vi "WSVCAP SHL Host LL Interface Core.vi"(0 "Message In":string, 11 "error in":errorcluster, 12 "Log (T)":bool=TRUE, 13 "Function":T5, 14 "FPGA":T1) -> (3 "System":T2={"Settings"={"I2C Slave Address"=144, "I2C Clock Rate (Hz)"=20.0, "SPI Clock Rate (Hz)"=50000.0, "RFFE Slave Address"=255, "RFFE Clock Rate (Hz)"=20.0, "Simulate FPGA"=TRUE, "C1 Cap DAC Default"=165, "C2 Cap DAC Default"=165, "C3 Cap DAC Default"=134}, "FPGA Resource"="", "Online"=FALSE, "I2C Wait Ticks"=0, "SPI Wait Ticks"=0, "RFFE Wait Ticks"=0, "FPGA VI Reference (FPGA Mode)"=refnum, "FPGA VI Reference (Sim Mode)"=refnum} {"Settings"."C3 Cap DAC Default" format="0x%02x"; "Settings"."C2 Cap DAC Default" format="0x%02x"; "Settings"."C1 Cap DAC Default" format="0x%02x"; "Settings"."RFFE Clock Rate (Hz)" format="%.0f Hz"; "Settings"."RFFE Slave Address" format="0x%02x"; "Settings"."I2C Clock Rate (Hz)" format="%.0f Hz"; "Settings"."SPI Clock Rate (Hz)" format="%.0f Hz"; "Settings"."I2C Slave Address" format="0x%02x"}, 4 "Message Out":string, 15 "error out":errorcluster)   [LabVIEW 2012]
uses:
  Type Defs/WSVCAP SHL Function Enum.ctl
  Type Defs/WSVCAP SHL Core System Cluster.ctl
  Type Defs/WSVCAP SHL I2C Settings Cluster.ctl
  Type Defs/WSVCAP SHL FPGA VI Reference.ctl
  Type Defs/WSVCAP SHL I2C FPGA Enum.ctl
  user.lib/Configuration Files/Type Defs/CFG File Operation Enum.ctl
  Type Defs/WSVCAP SHL Top Level Control Operation Enum.ctl
  Type Defs/WSVCAP SHL Top Level Control Enum.ctl
  <vilib>/FPGAPlugInAG/PXI-7813R/niLvFpga_Open_PXI-7813R.vi
  <vilib>/FPGAPlugInAG/PXI-7813R/niLvFpga_Reset_PXI-7813R.vi
  <vilib>/FPGAPlugInAG/PXI-7813R/niLvFpga_Run_PXI-7813R.vi
  <vilib>/FPGAPlugInAG/PXI-7813R/niLvFpga_Abort_PXI-7813R.vi
  <vilib>/FPGAPlugInAG/PXI-7813R/niLvFpga_Close_PXI-7813R.vi
  <vilib>/rvi/interface/nirviOpenFPGA/nirviOpenFPGA.xnode
  FPGA Bitfiles/WSVCAPShell_WiSpryFPGA1_WSVCAPSHLFPGATLT_acCLp6kl0Ls.lvbitx
  <vilib>/rvi/interface/nirviMethod/nirviMethod.xnode
  <vilib>/rvi/interface/nirviCloseFPGA/nirviCloseFPGA.xnode
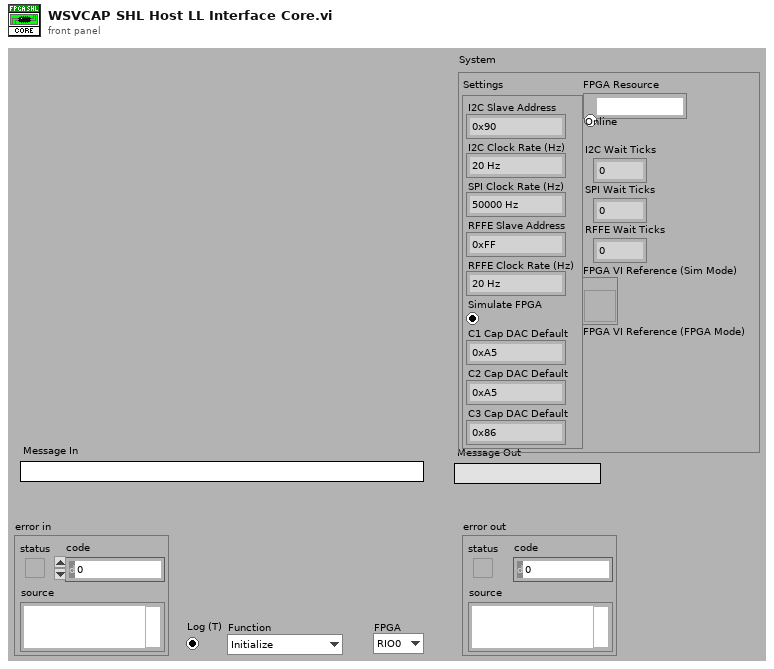
[diagram p1: front panel]
types:
  T1 = typedef "WSVCAP SHL I2C FPGA Enum.ctl" = enum16{"RIO0", "RIO1"}
  T2 = typedef "WSVCAP SHL Core System Cluster.ctl" = cluster{"Settings":T3, "FPGA Resource":tag, "Online":bool, "I2C Wait Ticks":u32, "SPI Wait Ticks":u32, "RFFE Wait Ticks":u32, "FPGA VI Reference (FPGA Mode)":T4, "FPGA VI Reference (Sim Mode)":refnum<vi>}
  T3 = typedef "WSVCAP SHL I2C Settings Cluster.ctl" = cluster{"I2C Slave Address":u8, "I2C Clock Rate (Hz)":dbl, "SPI Clock Rate (Hz)":dbl, "RFFE Slave Address":u8, "RFFE Clock Rate (Hz)":dbl, "Simulate FPGA":bool, "C1 Cap DAC Default":u8, "C2 Cap DAC Default":u8, "C3 Cap DAC Default":u8}
  T4 = typedef "WSVCAP SHL FPGA VI Reference.ctl" = refnum<k20>
  T5 = typedef "WSVCAP SHL Function Enum.ctl" = enum16{"Initialize", "Configure I2C", "Configure RFFE", "Write I2C", "Read I2C", "Write RFFE", "Read RFFE", "Start RFFE Cycle", "Stop RFFE Cycle", "Get Status", "Close"}
  T6 = typedef "WSVCAP SHL Top Level Control Operation Enum.ctl" = enum16{"Initialize", "Set Control", "Read Control", "Close"}
  T7 = typedef "CFG File Operation Enum.ctl" = enum16{"Read", "Write", "Copy", "Edit"}
  T8 = enum32{"Invalid", "Standard", "Closed", "Hidden", "Minimized", "Maximized"}
  T9 = typedef "WSVCAP SHL Top Level Control Enum.ctl" = enum16{"Start", "Cmd", "Transaction", "Wait Ticks", "Socket Mask", "UUT Set", "Slave Address", "Sub Address", "Bytes to Write", "Bytes to Read", "Write Data", "Write Flag", "Read Data", "Read Flag", "Ack Read", "Read Status Flag", "Ack Read Status", "Status", "Cycle Count", "Stop Cycle", "Exit"}
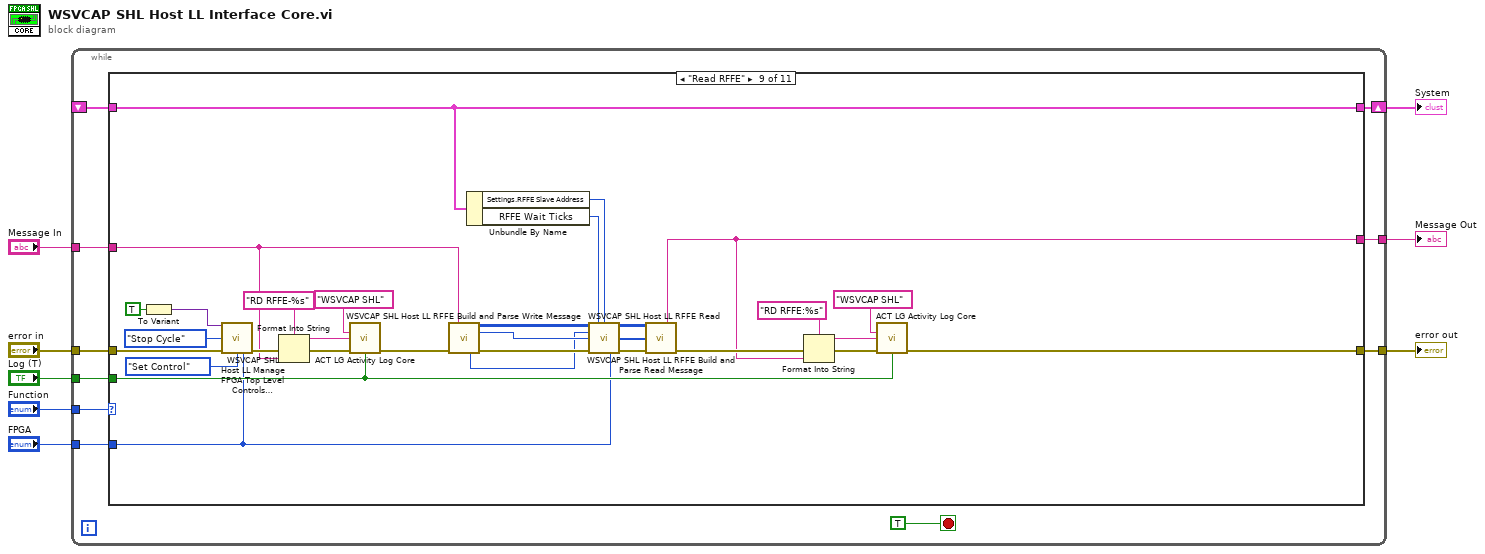
[diagram p0: block diagram]
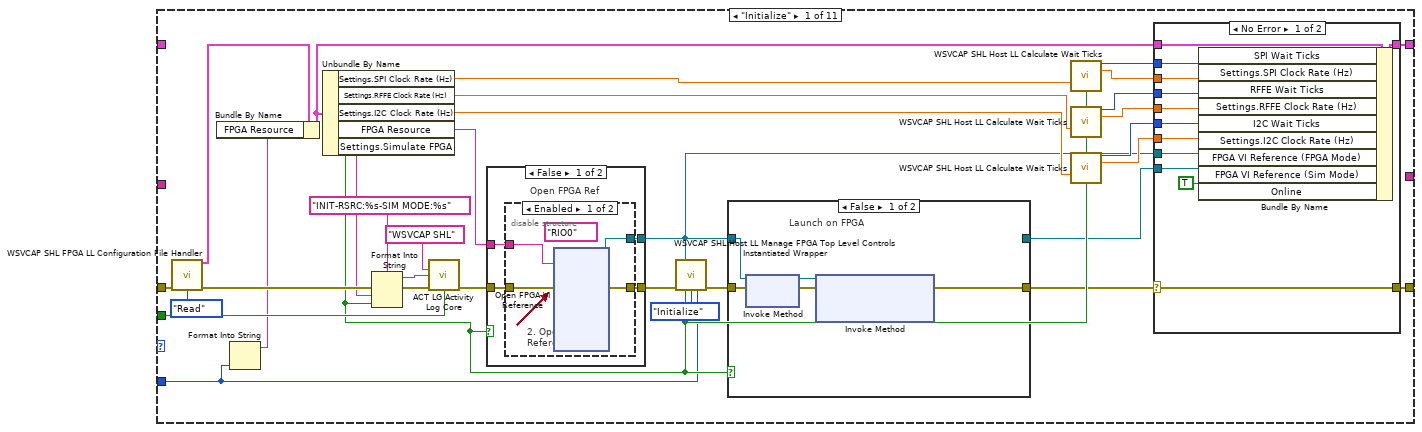
[diagram p2: hidden frame]
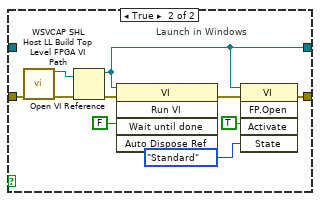
[diagram p5: hidden frame]
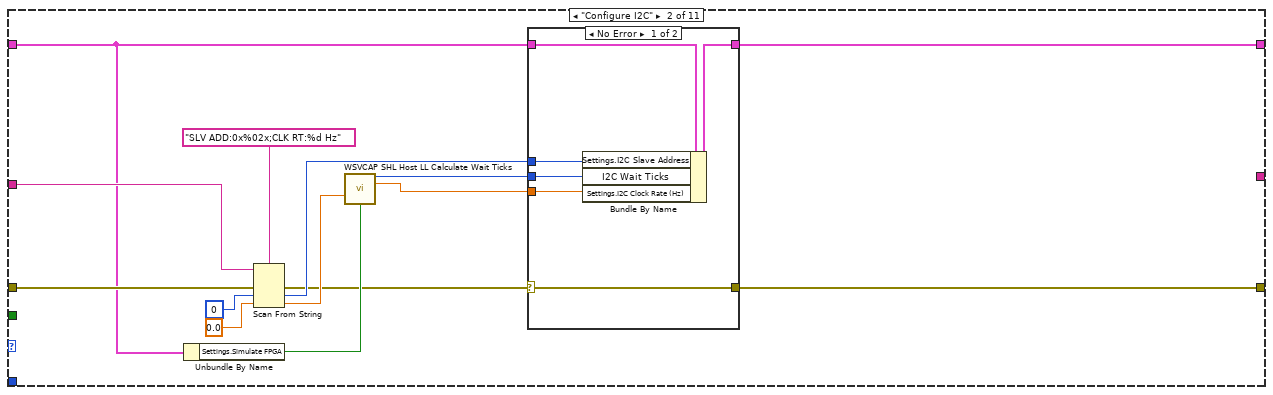
[diagram p7: hidden frame]
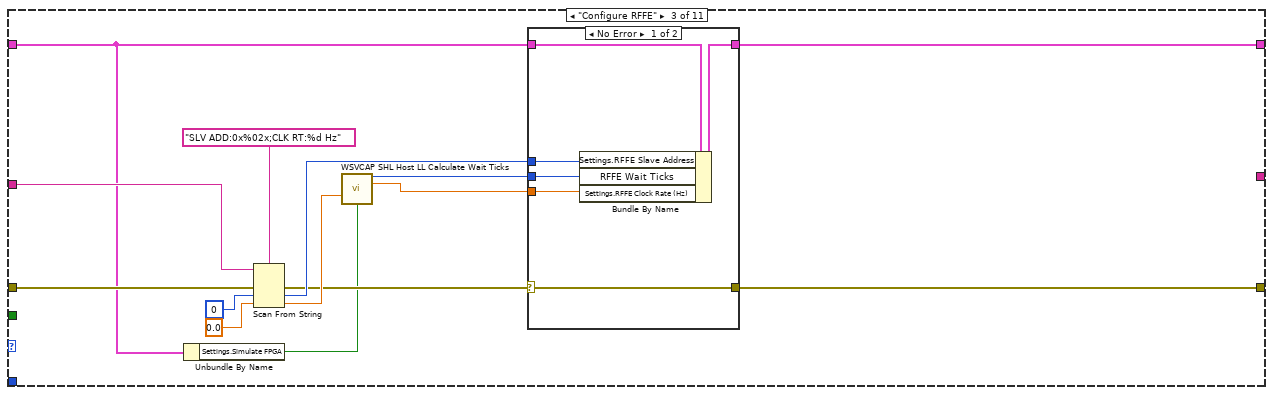
[diagram p9: hidden frame]
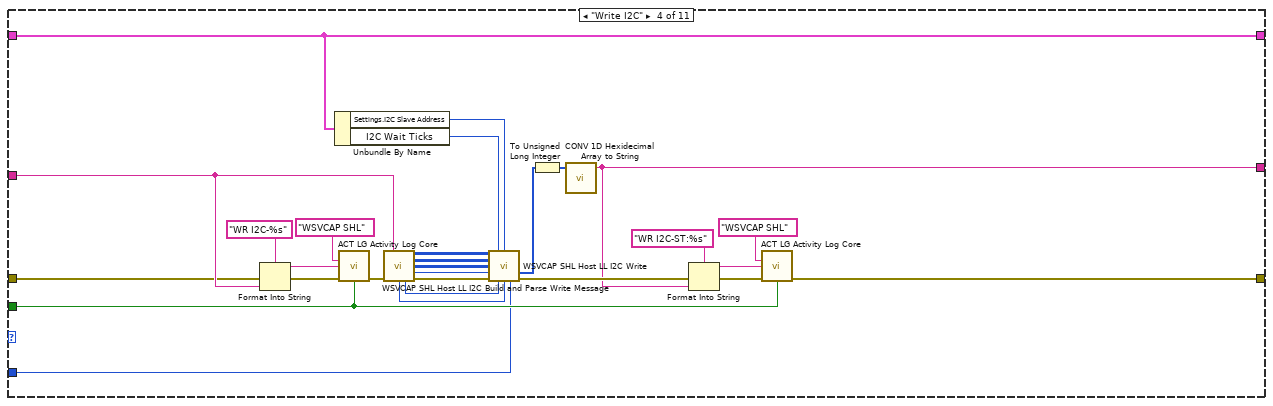
[diagram p11: hidden frame]
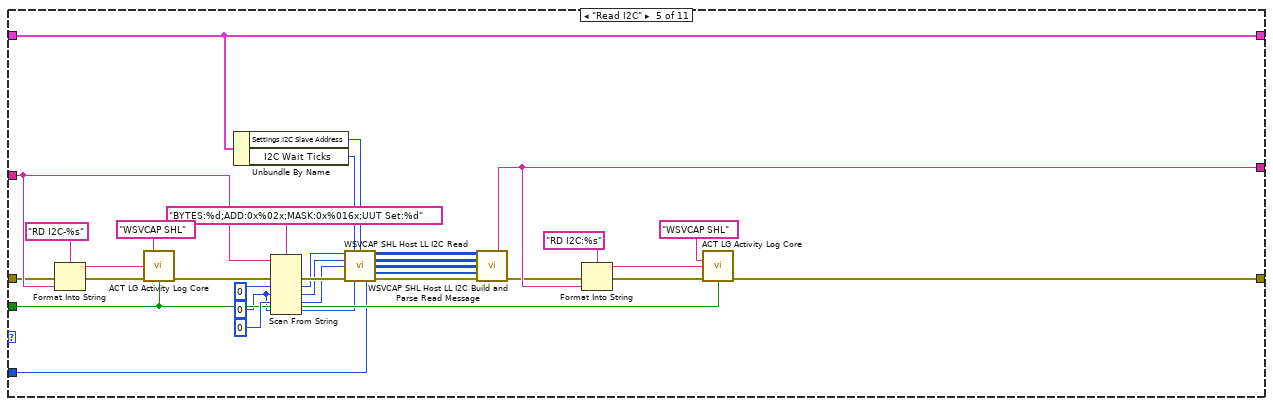
[diagram p12: hidden frame]
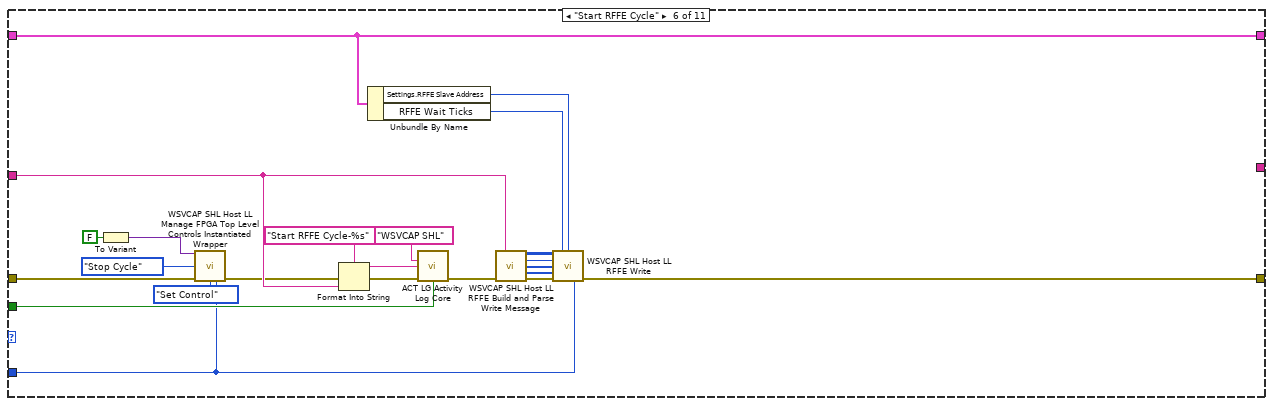
[diagram p13: hidden frame]
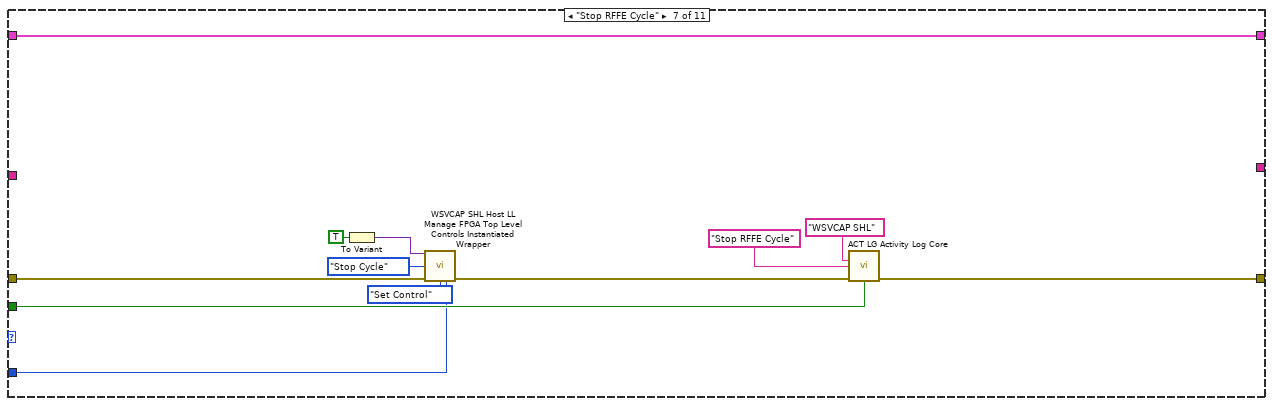
[diagram p14: hidden frame]
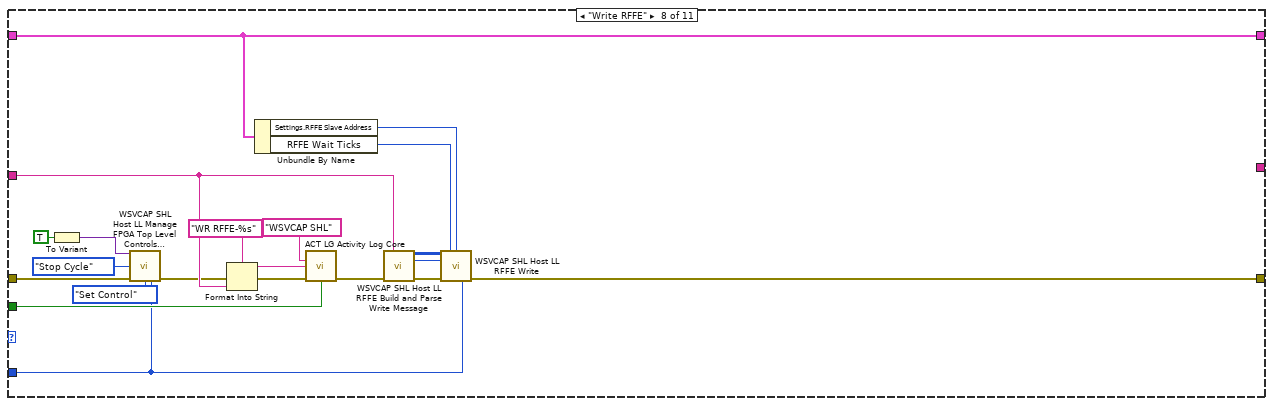
[diagram p15: hidden frame]
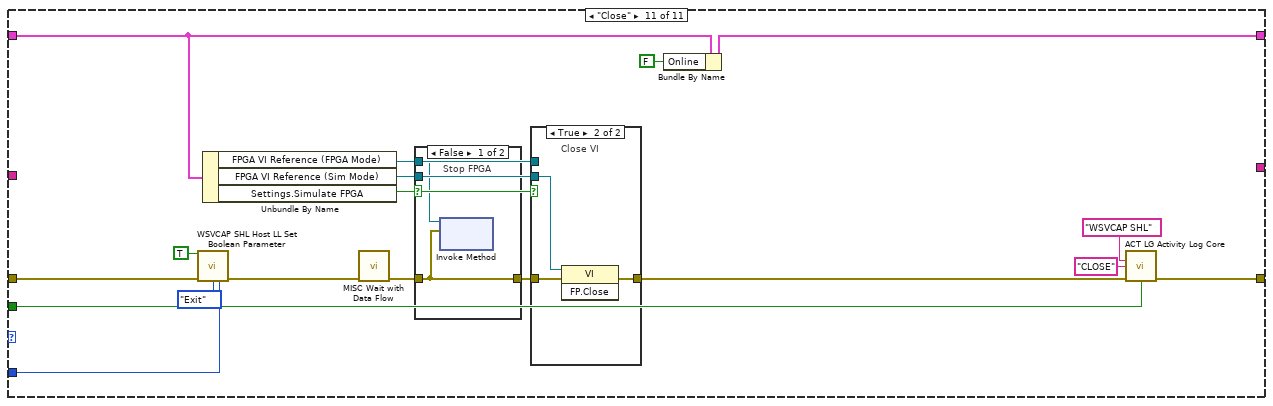
[diagram p17: hidden frame]
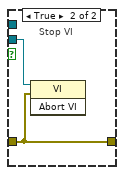
[diagram p18: hidden frame]
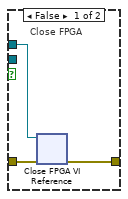
[diagram p19: hidden frame]
diagram:
  n1 = while {
    tunnel: "Function" -> [w17]
    tunnel: "error in" -> [w16]
    tunnel: "Message In" -> [w15]
    tunnel: [w9] -> w5
    shift-right: [w12] -> w4
    shift-left: _ -> [w14]
    tunnel: [w13] -> w3
    tunnel: "Log (T)" -> [w11]
    tunnel: "FPGA" -> [w10]
    stop <- TRUE ("stop") stop-if-true
    n2 = case shown="\"Read RFFE\"" w17 {
      tunnel: w16 -> [w46 w101 w123 w152 w176 w200 w221 w237 w262 w282 w298]
      tunnel: w15 -> [_ w100 w122 w153 w177 w210 _ w243 w255 _ _]
      tunnel: [w49 w102 w124 w154 w173 w208 w227 w232 w269 w282 w295] -> w9
      tunnel: [w50 w103 w125 w140 w169 w198 w229 w234 w260 w283 w301] -> w12
      tunnel: w14 -> [_ w96 w118 w140 w169 w198 w229 w234 w260 w283 w289]
      tunnel: [_ _ _ w144 w178 _ _ _ w268 _ _] -> w13
      tunnel: w11 -> [w39 _ _ w141 w170 w209 w226 w242 w267 _ w293]
      tunnel: w10 -> [w22 _ _ w134 w162 w195 w220 w230 w251 _ w292]
      frame "Initialize" {
        n3 = call "WSVCAP SHL FPGA LL Configuration File Handler.vi"("Error In (no error)"=w46, "Operation"=CFG_File_Operation_Enum."Read") -> ("Object Cluster Out"=w20:T2, "Error Out"=w44:errorcluster)  [unwired: 11 in, 1 out]
        n4 = Format Into String(w22) -> (resulting string=w21:string)  [unwired: 3 in, 1 out]
        n5 = Bundle By Name(cluster=w20, "FPGA Resource"=w21) -> (w19:T2)
        n6 = Unbundle By Name(w19) -> ("Settings.SPI Clock Rate (Hz)"=w34:dbl, "Settings.RFFE Clock Rate (Hz)"=w37:dbl, "Settings.I2C Clock Rate (Hz)"=w41:dbl, "FPGA Resource"=w28:tag, "Settings.Simulate FPGA"=w27:bool)
        n7 = Format Into String(format string="INIT-RSRC:%s-SIM MODE:%s", error in=w44, w28, w27) -> (resulting string=w45:string, error out=w43:errorcluster)  [unwired: 1 in]
        n8 = call "ACT LG Activity Log Core.vi"("Source"="WSVCAP SHL", "Log Line"=w45, "Error In (no error)"=w43, "Log (T)"=w39) -> ("Error Out"=w26:errorcluster)  [unwired: 10 in, 1 out]
        n9 = case shown="False" w27 {
          tunnel: [w54 w60] -> w31
          tunnel: w26 -> [w53 w60]
          tunnel: [w52 _] -> w23
          tunnel: w28 -> [w51 _]
          frame False {
            # "Open FPGA Ref"
            n10 = disable-structure shown="Enabled" {
              disable-tunnel: w53 -> [w58 w59]
              disable-tunnel: [w57 w59] -> w54
              disable-tunnel: [w56 _] -> w52
              disable-tunnel: w51 -> [w55 _]
              frame Enabled {
                (unwired) tag "RIO0" ("resource name")
                # "2. Open FPGA VI Reference"
                n11 = xnode "Open FPGA VI Reference"("error in"=w58, "resource name"=w55) -> ("FPGA VI Reference Out"=w56:refnum<k20>, "error out"=w57:errorcluster)
              }
              frame Disabled {
              }
            }
          }
          frame True {
            # "Simulate FPGA"
          }
        }
        n12 = call "WSVCAP SHL Host LL Manage FPGA Top Level Controls Instantiated Wrapper.vi"("FPGA VI Reference (Init Only)"=w23, "error in (no error)"=w31, "Simulate FPGA (Init Only)"=w27, "Operation"=WSVCAP_SHL_Top_Level_Control_Operation_Enum."Initialize", "FPGA"=w22) -> ("error out"=w29:errorcluster)  [unwired: 9 in, 1 out]
        n13 = case shown="False" w27 {
          tunnel: w29 -> [w64 w68]
          tunnel: [w63 w71] -> w25
          tunnel: w23 -> [w61 _]
          tunnel: [_ w72] -> w24
          frame False {
            # "Launch on FPGA"
            n14 = xnode "Invoke Method"("FPGA VI Reference In"=w61, "error in"=w64) -> ("FPGA VI Reference Out"=w62:refnum<k20>, "error out"=w65:errorcluster)
            n15 = xnode "Invoke Method"("FPGA VI Reference In"=w62, "error in"=w65) -> ("error out"=w63:errorcluster)  [unwired: 1 in, 1 out]
          }
          frame True {
            # "Launch in Windows"
            n16 = call "WSVCAP SHL Host LL Build Top Level FPGA VI Path.vi"("Error In (no error)"=w68) -> ("Top Level FPGA VI Path"=w66:path, "Error Out"=w67:errorcluster)  [unwired: 13 in]
            n17 = Open VI Reference(vi path=w66, error in (no error)=w67) -> (vi reference=w72:refnum<vi>, error out=w75:errorcluster)  [unwired: 4 in]
            n18 = invoke class="VI" method="Run VI"(reference=w72, error in=w75, "Wait until done"=FALSE ("Wait Until Done")) -> (error out=w73:errorcluster)  [unwired: 2 in, 4 out]
            n19 = invoke class="VI" method="FP.Open"(reference=w72, error in=w73, "Activate"=TRUE ("Activate?"), "State"=T8."Standard" ("Front Panel Window:State")) -> (error out=w71:errorcluster)  [unwired: 1 in, 4 out]
          }
        }
        n20 = call "WSVCAP SHL Host LL Calculate Wait Ticks.vi"("Clock Rate (Hz)"=w34, "Simulate FPGA"=w27) -> ("Wait Ticks"=w33:u32, "Actual Rate (Hz)"=w32:dbl)  [unwired: 12 in]
        n21 = call "WSVCAP SHL Host LL Calculate Wait Ticks.vi"("Clock Rate (Hz)"=w37, "Simulate FPGA"=w27) -> ("Wait Ticks"=w36:u32, "Actual Rate (Hz)"=w35:dbl)  [unwired: 12 in]
        n22 = call "WSVCAP SHL Host LL Calculate Wait Ticks.vi"("Clock Rate (Hz)"=w41, "Simulate FPGA"=w27) -> ("Wait Ticks"=w38:u32, "Actual Rate (Hz)"=w48:dbl)  [unwired: 12 in]
        n23 = case shown="No Error" w25 {
          selector: w25 -> [w85 w88]
          tunnel: w19 -> [w87 w89]
          tunnel: [w86 w89] -> w50
          tunnel: [w85 w88] -> w49
          tunnel: w48 -> [w84 _]
          tunnel: w38 -> [w83 _]
          tunnel: w36 -> [w82 _]
          tunnel: w35 -> [w81 _]
          tunnel: w33 -> [w80 _]
          tunnel: w32 -> [w79 _]
          tunnel: w23 -> [w77 _]
          tunnel: w24 -> [w76 _]
          frame No Error {
            n24 = Bundle By Name(cluster=w87, "SPI Wait Ticks"=w80, "Settings.SPI Clock Rate (Hz)"=w79, "RFFE Wait Ticks"=w82, "Settings.RFFE Clock Rate (Hz)"=w81, "I2C Wait Ticks"=w83, "Settings.I2C Clock Rate (Hz)"=w84, "FPGA VI Reference (FPGA Mode)"=w77, "FPGA VI Reference (Sim Mode)"=w76, "Online"=TRUE) -> (w86:T2)
          }
          frame Error {
          }
        }
      }
      frame "Configure I2C" {
        n25 = Unbundle By Name(w96) -> ("Settings.Simulate FPGA"=w95:bool)
        n26 = Scan From String(format string="SLV ADD:0x%02x;CLK RT:%d Hz", input string=w100, error in=w101, default 1=u8 0 ("I2C_Slave Address"), default 2=0.0 ("Clock Rate (Hz)")) -> (error out=w90:errorcluster, output 1=w97:u8, output 2=w93:dbl)  [unwired: 1 in, 2 out]
        n27 = call "WSVCAP SHL Host LL Calculate Wait Ticks.vi"("Clock Rate (Hz)"=w93, "Simulate FPGA"=w95) -> ("Wait Ticks"=w91:u32, "Actual Rate (Hz)"=w92:dbl)  [unwired: 12 in]
        n28 = case shown="No Error" w90 {
          selector: w90 -> [w107 w110]
          tunnel: w96 -> [w109 w111]
          tunnel: [w108 w111] -> w103
          tunnel: [w107 w110] -> w102
          tunnel: w97 -> [w106 _]
          tunnel: w92 -> [w105 _]
          tunnel: w91 -> [w104 _]
          frame No Error {
            n29 = Bundle By Name(cluster=w109, "Settings.I2C Slave Address"=w106, "I2C Wait Ticks"=w104, "Settings.I2C Clock Rate (Hz)"=w105) -> (w108:T2)
          }
          frame Error {
          }
        }
      }
      frame "Configure RFFE" {
        n30 = Unbundle By Name(w118) -> ("Settings.Simulate FPGA"=w112:bool)
        n31 = Scan From String(format string="SLV ADD:0x%02x;CLK RT:%d Hz", input string=w122, error in=w123, default 1=u8 0 ("I2C_Slave Address"), default 2=0.0 ("Clock Rate (Hz)")) -> (error out=w113:errorcluster, output 1=w119:u8, output 2=w116:dbl)  [unwired: 1 in, 2 out]
        n32 = call "WSVCAP SHL Host LL Calculate Wait Ticks.vi"("Clock Rate (Hz)"=w116, "Simulate FPGA"=w112) -> ("Wait Ticks"=w115:u32, "Actual Rate (Hz)"=w114:dbl)  [unwired: 12 in]
        n33 = case shown="No Error" w113 {
          selector: w113 -> [w129 w132]
          tunnel: w118 -> [w131 w133]
          tunnel: [w130 w133] -> w125
          tunnel: [w129 w132] -> w124
          tunnel: w119 -> [w128 _]
          tunnel: w114 -> [w127 _]
          tunnel: w115 -> [w126 _]
          frame No Error {
            n34 = Bundle By Name(cluster=w131, "Settings.RFFE Slave Address"=w128, "RFFE Wait Ticks"=w126, "Settings.RFFE Clock Rate (Hz)"=w127) -> (w130:T2)
          }
          frame Error {
          }
        }
      }
      frame "Write I2C" {
        n35 = Format Into String(format string="WR I2C-%s", error in=w152, w153) -> (resulting string=w149:string, error out=w151:errorcluster)  [unwired: 1 in]
        n36 = Unbundle By Name(w140) -> ("Settings.I2C Slave Address"=w136:u8, "I2C Wait Ticks"=w139:u32)
        n37 = call "ACT LG Activity Log Core.vi"("Source"="WSVCAP SHL", "Log Line"=w149, "Error In (no error)"=w151, "Log (T)"=w141) -> ("Error Out"=w156:errorcluster)  [unwired: 10 in, 1 out]
        n38 = call "WSVCAP SHL Host LL I2C Build and Parse Write Message.vi"("Message In"=w153, "error in"=w156) -> ("C1 Write Data Out [DUT Ordered]"=w160:u8[][], "C2 Write Data Out [DUT Ordered]"=w158:u8[][], "C3 Write Data Out [DUT Ordered]"=w138:u8[][], "Socket Mask [U64] Out"=w159:u64, "UUT Set (0/1) Out"=w135:u8, "Sub Address Out"=w137:u8, "error out"=w161:errorcluster)  [unwired: 6 in, 1 out]
        n39 = call "WSVCAP SHL Host LL I2C Write.vi"("C1 Data Out [DUT Ordered]"=w160, "Wait Ticks"=w139, "Slave Address"=w136, "C2 Data Out [DUT Ordered]"=w158, "C3 Data Out [DUT Ordered]"=w138, "Socket Mask [U64]"=w159, "error in"=w161, "Sub Address"=w137, "UUT Set (0/1)"=w135, "FPGA"=w134) -> ("Status"=w146:u8[], "error out"=w148:errorcluster)  [unwired: 4 in]
        n40 = To Unsigned Long Integer(number=w146) -> (unsigned 32bit integer=w145:u32[])
        n41 = call "CONV 1D Hexidecimal Array to String.vi"("1-D Hexidecimal"=w145) -> ("String"=w144:string)  [unwired: 8 in]
        n42 = Format Into String(format string="WR I2C-ST:%s", error in=w148, w144) -> (resulting string=w142:string, error out=w147:errorcluster)  [unwired: 1 in]
        n43 = call "ACT LG Activity Log Core.vi"("Source"="WSVCAP SHL", "Log Line"=w142, "Error In (no error)"=w147, "Log (T)"=w141) -> ("Error Out"=w154:errorcluster)  [unwired: 10 in, 1 out]
      }
      frame "Read I2C" {
        w164 = u8 0 ("Sub Address [U8]")
        n44 = Format Into String(format string="RD I2C-%s", error in=w176, w177) -> (resulting string=w182:string, error out=w184:errorcluster)  [unwired: 1 in]
        n45 = call "ACT LG Activity Log Core.vi"("Source"="WSVCAP SHL", "Log Line"=w182, "Error In (no error)"=w184, "Log (T)"=w170) -> ("Error Out"=w175:errorcluster)  [unwired: 10 in, 1 out]
        n46 = Unbundle By Name(w169) -> ("Settings.I2C Slave Address"=w165:u8, "I2C Wait Ticks"=w168:u32)
        n47 = Scan From String(format string="BYTES:%d;ADD:0x%02x;MASK:0x%016x;UUT Set:%d", input string=w177, error in=w175, default 1=u8 0 ("Bytes to Read"), default 2=w164, default 3=u64 0 ("Socket Mask [U32]"), default 4=w164) -> (error out=w194:errorcluster, output 1=w191:u8, output 2=w189:u8, output 3=w190:u64, output 4=w163:u8)  [unwired: 1 in, 2 out]
        n48 = call "WSVCAP SHL Host LL I2C Read.vi"("Bytes to Read"=w191, "Wait Ticks"=w168, "Slave Address"=w165, "Sub Address [U8]"=w189, "Socket Mask [U64]"=w190, "error in"=w194, "UUT Set (0/1)"=w163, "FPGA"=w162) -> ("C1:1-18 Read Data [DUT Ordered]"=w187:u8[][], "C2:1-18 Read Data [DUT Ordered]"=w186:u8[][], "C3:1-18 Read Data [DUT Ordered]"=w167:u8[][], "Status"=w166:u8[], "error out"=w188:errorcluster)  [unwired: 3 in]
        n49 = call "WSVCAP SHL Host LL I2C Build and Parse Read Message.vi"("C1 Read Data In"=w187, "C2 Read Data"=w186, "C3 Read Data"=w167, "Status In"=w166, "error in"=w188) -> ("Message Out"=w178:string, "error out"=w174:errorcluster)  [unwired: 5 in, 4 out]
        n50 = Format Into String(format string="RD I2C:%s", error in=w174, w178) -> (resulting string=w179:string, error out=w181:errorcluster)  [unwired: 1 in]
        n51 = call "ACT LG Activity Log Core.vi"("Source"="WSVCAP SHL", "Log Line"=w179, "Error In (no error)"=w181, "Log (T)"=w170) -> ("Error Out"=w173:errorcluster)  [unwired: 10 in, 1 out]
      }
      frame "Start RFFE Cycle" {
        n52 = To Variant(anything=FALSE ("Cycle (F:Write/Read - T:Write Only - No Read)")) -> (Variant=w205:variant)
        n53 = call "WSVCAP SHL Host LL Manage FPGA Top Level Controls Instantiated Wrapper.vi"("Value In"=w205, "FPGA Top Level Control"=WSVCAP_SHL_Top_Level_Control_Enum."Stop Cycle", "error in (no error)"=w200, "Operation"=WSVCAP_SHL_Top_Level_Control_Operation_Enum."Set Control", "FPGA"=w195) -> ("error out"=w199:errorcluster)  [unwired: 9 in, 1 out]
        n54 = Format Into String(format string="Start RFFE Cycle-%s", error in=w199, w210) -> (resulting string=w212:string, error out=w214:errorcluster)  [unwired: 1 in]
        n55 = Unbundle By Name(w198) -> ("Settings.RFFE Slave Address"=w196:u8, "RFFE Wait Ticks"=w197:u32)
        n56 = call "ACT LG Activity Log Core.vi"("Source"="WSVCAP SHL", "Log Line"=w212, "Error In (no error)"=w214, "Log (T)"=w209) -> ("Error Out"=w211:errorcluster)  [unwired: 10 in, 1 out]
        n57 = call "WSVCAP SHL Host LL RFFE Build and Parse Write Message.vi"("Message In"=w210, "error in"=w211) -> ("Write Data Out [DUT Ordered]"=w216:u8[][], "Socket Mask [U16] Out"=w203:u64, "Cycle CMD Lengths Out (bits)"=w202:u8[], "Cycle CMD Delay Out (ticks)"=w201:u32[], "error out"=w217:errorcluster)  [unwired: 7 in, 2 out]
        n58 = call "WSVCAP SHL Host LL RFFE Write.vi"("RTFFE Data [DUT Ordered]"=w216, "Wait Ticks"=w197, "Slave Address"=w196, "Socket Mask"=w203, "Cycle CMD Lengths Out (bits)"=w202, "Cycle CMD Delay Out (ticks)"=w201, "error in"=w217, "FPGA"=w195) -> ("error out"=w208:errorcluster)  [unwired: 6 in, 1 out]
      }
      frame "Stop RFFE Cycle" {
        n59 = To Variant(anything=TRUE ("Cycle (F:Write/Read - T:Write Only - No Read)")) -> (Variant=w222:variant)
        n60 = call "WSVCAP SHL Host LL Manage FPGA Top Level Controls Instantiated Wrapper.vi"("Value In"=w222, "FPGA Top Level Control"=WSVCAP_SHL_Top_Level_Control_Enum."Stop Cycle", "error in (no error)"=w221, "Operation"=WSVCAP_SHL_Top_Level_Control_Operation_Enum."Set Control", "FPGA"=w220) -> ("error out"=w218:errorcluster)  [unwired: 9 in, 1 out]
        n61 = call "ACT LG Activity Log Core.vi"("Source"="WSVCAP SHL", "Log Line"="Stop RFFE Cycle" ("format string"), "Error In (no error)"=w218, "Log (T)"=w226) -> ("Error Out"=w227:errorcluster)  [unwired: 10 in, 1 out]
      }
      frame "Write RFFE" {
        n62 = To Variant(anything=TRUE ("Cycle (F:Write/Read - T:Write Only - No Read)")) -> (Variant=w239:variant)
        n63 = call "WSVCAP SHL Host LL Manage FPGA Top Level Controls Instantiated Wrapper.vi"("Value In"=w239, "FPGA Top Level Control"=WSVCAP_SHL_Top_Level_Control_Enum."Stop Cycle", "error in (no error)"=w237, "Operation"=WSVCAP_SHL_Top_Level_Control_Operation_Enum."Set Control", "FPGA"=w230) -> ("error out"=w236:errorcluster)  [unwired: 9 in, 1 out]
        n64 = Format Into String(format string="WR RFFE-%s", error in=w236, w243) -> (resulting string=w245:string, error out=w247:errorcluster)  [unwired: 1 in]
        n65 = Unbundle By Name(w234) -> ("Settings.RFFE Slave Address"=w231:u8, "RFFE Wait Ticks"=w233:u32)
        n66 = call "ACT LG Activity Log Core.vi"("Source"="WSVCAP SHL", "Log Line"=w245, "Error In (no error)"=w247, "Log (T)"=w242) -> ("Error Out"=w244:errorcluster)  [unwired: 10 in, 1 out]
        n67 = call "WSVCAP SHL Host LL RFFE Build and Parse Write Message.vi"("Message In"=w243, "error in"=w244) -> ("Write Data Out [DUT Ordered]"=w249:u8[][], "Socket Mask [U16] Out"=w235:u64, "error out"=w250:errorcluster)  [unwired: 7 in, 4 out]
        n68 = call "WSVCAP SHL Host LL RFFE Write.vi"("RTFFE Data [DUT Ordered]"=w249, "Wait Ticks"=w233, "Slave Address"=w231, "Socket Mask"=w235, "error in"=w250, "FPGA"=w230) -> ("error out"=w232:errorcluster)  [unwired: 8 in, 1 out]
      }
      frame "Read RFFE" {
        n69 = To Variant(anything=TRUE ("Cycle (F:Write/Read - T:Write Only - No Read)")) -> (Variant=w264:variant)
        n70 = call "WSVCAP SHL Host LL Manage FPGA Top Level Controls Instantiated Wrapper.vi"("Value In"=w264, "FPGA Top Level Control"=WSVCAP_SHL_Top_Level_Control_Enum."Stop Cycle", "error in (no error)"=w262, "Operation"=WSVCAP_SHL_Top_Level_Control_Operation_Enum."Set Control", "FPGA"=w251) -> ("error out"=w261:errorcluster)  [unwired: 9 in, 1 out]
        n71 = Format Into String(format string="RD RFFE-%s", error in=w261, w255) -> (resulting string=w274:string, error out=w276:errorcluster)  [unwired: 1 in]
        n72 = call "ACT LG Activity Log Core.vi"("Source"="WSVCAP SHL", "Log Line"=w274, "Error In (no error)"=w276, "Log (T)"=w267) -> ("Error Out"=w257:errorcluster)  [unwired: 10 in, 1 out]
        n73 = call "WSVCAP SHL Host LL RFFE Build and Parse Write Message.vi"("Message In"=w255, "error in"=w257) -> ("Write Data Out [DUT Ordered]"=w254:u8[][], "Socket Mask [U16] Out"=w253:u64, "Byte Count"=w252:u8, "error out"=w256:errorcluster)  [unwired: 7 in, 3 out]
        n74 = Unbundle By Name(w260) -> ("Settings.RFFE Slave Address"=w258:u8, "RFFE Wait Ticks"=w259:u32)
        n75 = call "WSVCAP SHL Host LL RFFE Read.vi"("RFFE Data [DUT Ordered]"=w254, "Wait Ticks"=w259, "Slave Address"=w258, "Bytes to Read"=w252, "Socket Mask [U64]"=w253, "error in"=w256, "FPGA"=w251) -> ("RFFE Read Data [DUT Ordered]"=w280:u8[][], "Status"=w279:u8[], "error out"=w281:errorcluster)  [unwired: 6 in]
        n76 = call "WSVCAP SHL Host LL RFFE Build and Parse Read Message.vi"("Write Data In"=w280, "Status In"=w279, "error in"=w281) -> ("Message Out"=w268:string, "error out"=w270:errorcluster)  [unwired: 9 in, 2 out]
        n77 = Format Into String(format string="RD RFFE:%s", error in=w270, w268) -> (resulting string=w271:string, error out=w273:errorcluster)  [unwired: 1 in]
        n78 = call "ACT LG Activity Log Core.vi"("Source"="WSVCAP SHL", "Log Line"=w271, "Error In (no error)"=w273, "Log (T)"=w267) -> ("Error Out"=w269:errorcluster)  [unwired: 10 in, 1 out]
      }
      frame "Get Status" {
      }
      frame "Close" {
        n79 = call "WSVCAP SHL Host LL Set Boolean Parameter.vi"("Boolean In"=TRUE ("Start"), "error in (no error)"=w298, "FPGA Top Level Control"=WSVCAP_SHL_Top_Level_Control_Enum."Exit", "FPGA"=w292) -> ("error out"=w285:errorcluster)  [unwired: 11 in]
        n80 = Unbundle By Name(w289) -> ("FPGA VI Reference (FPGA Mode)"=w288:T4, "FPGA VI Reference (Sim Mode)"=w287:refnum<vi>, "Settings.Simulate FPGA"=w286:bool)
        n81 = call "MISC Wait with Data Flow.vi"("Error In (no error)"=w285) -> ("Error Out"=w290:errorcluster)  [unwired: 8 in, 2 out]
        n82 = case shown="False" w286 {
          tunnel: w288 -> [w303 _]
          tunnel: w290 -> [w302 w304]
          tunnel: [w302 w304] -> w291
          tunnel: w287 -> [_ w305]
          frame False {
            # "Stop FPGA"
            n83 = xnode "Invoke Method"("FPGA VI Reference In"=w303, "error in"=w302) -> ()  [unwired: 2 out]
          }
          frame True {
            # "Stop VI"
            n84 = invoke class="VI" method="Abort VI"(reference=w305, error in=w304) -> ()  [unwired: 1 in, 3 out]
          }
        }
        n85 = case shown="True" w286 {
          tunnel: w291 -> [w308 w311]
          tunnel: w288 -> [w307 _]
          tunnel: [w306 w310] -> w284
          tunnel: w287 -> [_ w309]
          frame False {
            # "Close FPGA"
            n86 = xnode "Close FPGA VI Reference"("FPGA VI Reference In"=w307, "error in"=w308) -> ("error out"=w306:errorcluster)
          }
          frame True {
            # "Close VI"
            n87 = invoke class="VI" method="FP.Close"(reference=w309, error in=w311) -> (error out=w310:errorcluster)  [unwired: 1 in, 2 out]
          }
        }
        n88 = Bundle By Name(cluster=w289, "Online"=FALSE) -> (w301:T2)
        n89 = call "ACT LG Activity Log Core.vi"("Source"="WSVCAP SHL", "Log Line"="CLOSE", "Error In (no error)"=w284, "Log (T)"=w293) -> ("Error Out"=w295:errorcluster)  [unwired: 10 in, 1 out]
      }
    }
  }
  "error out" <- w5
  "Message Out" <- w3
  "System" <- w4
